vi "Set Defaults.vi"(11 "NewEntityTemplate in":refnum<class "NewEntityTemplate.lvclass">) -> (3 "NewEntityTemplate out":refnum<class "NewEntityTemplate.lvclass">)   [LabVIEW 2020, in "NewEntityTemplate.lvclass"]
uses:
  NewEntityTemplate.lvclass
  NewEntityTemplate.lvclass/NewEntityTemplate.ctl
  Conditum/Columns/Integer/Integer.lvclass
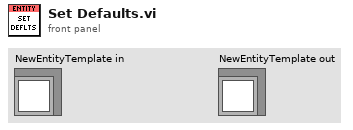
[diagram p1: front panel]
types:
  T1 = typedef "NewEntityTemplate.lvclass/Columns.ctl" = cluster{"<Placeholder>":refnum<class "Integer.lvclass">}
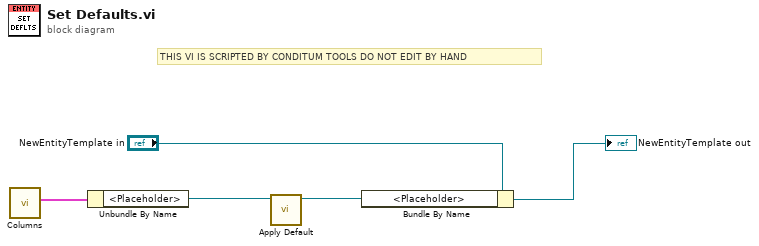
[diagram p0: block diagram]
diagram:
  # "THIS VI IS SCRIPTED BY CONDITUM TOOLS DO NOT EDIT BY HAND"
  n1 = call "Columns.vi"() -> ("Columns"=w5:T1)  [unwired: 11 in]
  n2 = Unbundle By Name(w5) -> ("<Placeholder>"=w4:refnum<class "Integer.lvclass">)
  n3 = call-dynamic "Apply Default.vi"("Integer in"=w4) -> ("Integer out"=w2:refnum<class "Integer.lvclass">)  [unwired: 10 in]
  n4 = Bundle By Name(cluster="NewEntityTemplate in", "<Placeholder>"=w2) -> (→"NewEntityTemplate out":refnum<class "NewEntityTemplate.lvclass">)
